vi "setStages.vi"(8 "error in (no error)":errorcluster, 10 "Stage":T1(ring), 11 "SingleToneRamp.lvclass in":refnum<class "SingleToneRamp.lvclass">) -> (0 "error out":errorcluster, 3 "SingleToneRamp.lvclass out":refnum<class "SingleToneRamp.lvclass">)   [LabVIEW 2009, in "Tools.lvlib" / "Scripting.lvlib" / "SingleToneRamp.lvclass"]
uses:
  SingleToneRamp.lvclass
  SingleTone.lvclass
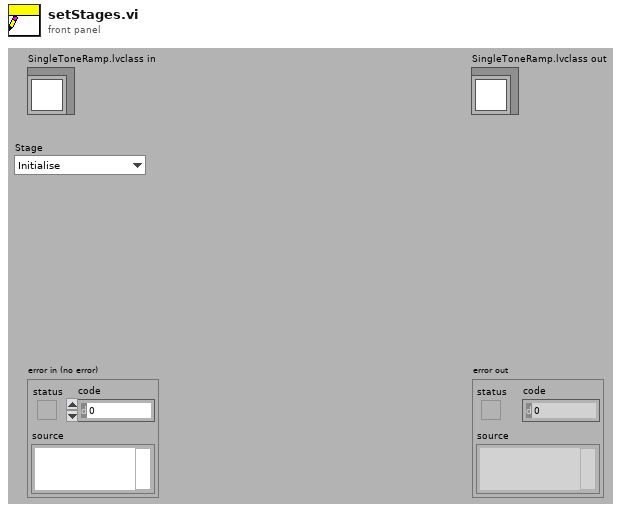
[diagram p1: front panel]
types:
  T1 = enum16{"Initialise", "MOT", "Molasses", "Optical Pumping", "Magnetic Trap", "RF Cooling", "Manipulation", "Switch Off", "Absorption Imaging", "Fluorscence Imaging", "Shut Down"}
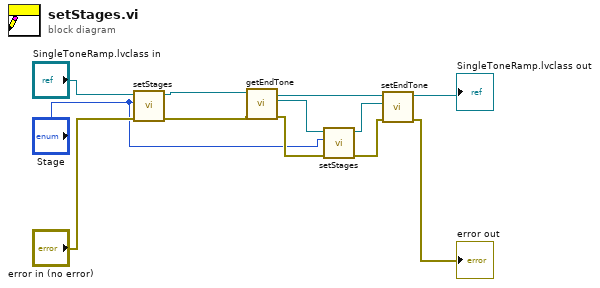
[diagram p0: block diagram]
diagram:
  n1 = call-parent "setStages.vi"("error in (no error)"="error in (no error)", "Stage"="Stage", "ScriptEvent.lvclass in"="SingleToneRamp.lvclass in") -> ("error out"=w2:errorcluster, "ScriptEvent.lvclass out"=w5:refnum<class "SingleToneRamp.lvclass">)  [unwired: 7 in]
  n2 = call "getEndTone.vi"("error in (no error)"=w2, "SingleToneRamp.lvclass in"=w5) -> ("error out"=w7:errorcluster, "endTone"=w9:refnum<class "SingleTone.lvclass">, "SingleToneRamp.lvclass out"=w10:refnum<class "SingleToneRamp.lvclass">)  [unwired: 7 in]
  n3 = call-parent "setStages.vi"("error in (no error)"=w7, "Stage"="Stage", "ScriptEvent.lvclass in"=w9) -> ("error out"=w6:errorcluster, "ScriptEvent.lvclass out"=w8:refnum<class "SingleTone.lvclass">)  [unwired: 7 in]
  n4 = call "setEndTone.vi"("error in (no error)"=w6, "EndTone"=w8, "SingleToneRamp.lvclass in"=w10) -> ("error out"=→"error out":errorcluster, "SingleToneRamp.lvclass out"=→"SingleToneRamp.lvclass out":refnum<class "SingleToneRamp.lvclass">)  [unwired: 7 in]
